vi "PPS TimeKeeper.vi"() -> ()   [LabVIEW 2016]
uses:
  LockPPS_State.ctl
  <vilib>/Platform/TimedLoop/XDataNode/timing_clust.ctl
  <vilib>/Platform/TimedLoop/XDataNode/nitl_modes.ctl
  <vilib>/Platform/TimedLoop/XDataNode/wakeup.ctl
  <vilib>/rvi/Emulation/niFpgaSctlEmulationGetInTimedLoop.vi
  <vilib>/rvi/Emulation/niFpgaEmulationReportErrorSimple.vi
  <vilib>/rvi/Emulation/niFpgaGetClockAttributes.vi
  <vilib>/rvi/Emulation/niFpgaCriticalErrorInLSC.vi
  <vilib>/rvi/eio/common/nirviEmuTemplateMethod_errors.vi
  <vilib>/Platform/TimedLoop/XDataNode/XDataNode.xnode
  <vilib>/eio/EIONode/EIONode.xnode
  <vilib>/rvi/FXPMathLib/basic elements/FxpDiscreteDelay/XNode/nifxpmath_DiscreteDelay.xnode
  <vilib>/Platform/TimedLoop/XDataNode/XDNodeRunTimeDep.lvlib
  <instrlib>/_niInstr/Basic Elements/v1/FPGA/niInstr Basic Elements v1 FPGA.lvlib
panel:
  out "state":T1
  in  "Dleay":u16=500
  out "PPS":u64
  in  "Period":u64=100000000 format="%.0p"
  in  "Lock":bool
  out "Time-ns":u64 format="%.0p"
  in  "Sync Counter Load Val":u64 format="%.0p"
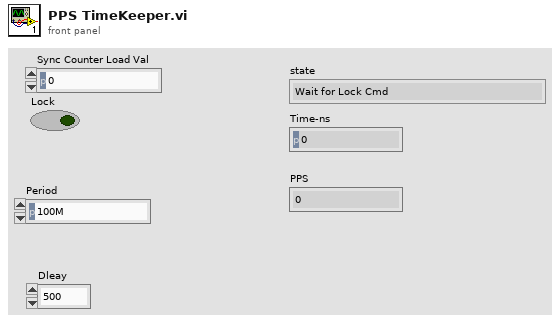
[diagram p1: front panel]
types:
  T1 = typedef "LockPPS_State.ctl" = enum16{"Wait for Lock Cmd", "Wait for PPS"}
  T2 = typedef "XDNodeRunTimeDep.lvlib/timing_clust.ctl" = cluster{"Expected End [f-1]":u64, "Actual End [f-1]":u64, "Finished Late? [f-1]":bool, "Expected End [i-1]":u64, "Actual End [i-1]":u64, "Finished Late? [i-1]":bool, "Expected Start [i]":u64, "Actual Start [i]":u64, "Expected Start [f]":u64, "Actual Start [f]":u64, "Source Name":string, "Structure Name":string, "Period":i64, "Deadline":i64, "Offset":i64, "Start":i64, "Priority":i32, "Timeout":i32, "Mode":T3, "Wakeup Reason":T4, "Error":errorcluster, "Source Type":string, "Secondary Source Type":string, "Global End Time":u64, "Global Start Time":u64, "Frame Duration":u64, "Iteration Duration":u64, "Assigned CPU":i32, "I/O Scan Engine Mode":u32}
  T3 = typedef "XDNodeRunTimeDep.lvlib/nitl_modes.ctl" = enum32{"No Change", "Process missed periods, maintain original phase", "Discard missed periods, maintain original phase", "Process missed periods, ignore original phase", "Discard missed periods, ignore original phase"}
  T4 = typedef "XDNodeRunTimeDep.lvlib/wakeup.ctl" = enum32{"Normal", "Aborted", "Asynchronous wakeup", "Timing source error", "Timed loop error", "Timeout"}
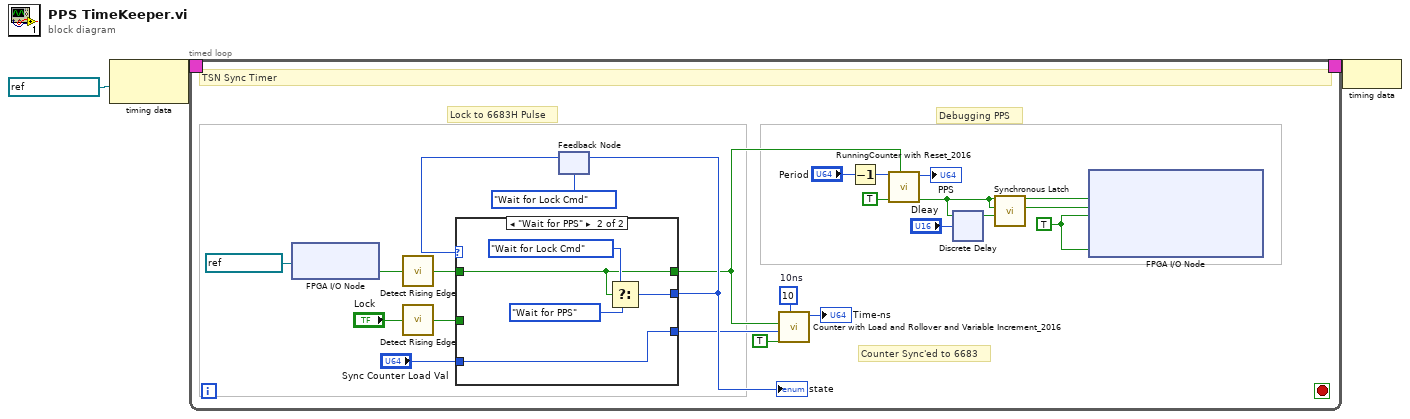
[diagram p0: block diagram]
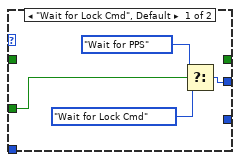
[diagram p2: hidden frame]
diagram:
  n1 = node-c288(refnum<k21> "PXIe_Clk100" ("Source Name")) -> (w3:T2)
  n2 = timed-loop {
    timing: w3 -> [_]
    timing-out: [_] -> w2
    stop <- _ stop-if-true
    w7 = u64 10  # 10ns
    w11 = TRUE ("Ethernet\\PFI0_OutEnable")
    # "Counter Sync'ed to 6683"
    # "Lock to 6683H Pulse"
    # "Debugging PPS"
    # "TSN Sync Timer"
    n3 = xnode "FPGA I/O Node"("FPGA I/O In"=refnum<k21> "PXI_Trig7") -> ("I/O Item"=w19:bool)  [unwired: 1 out]
    n4 = call <instrlib>:"Detect Rising Edge.vi"("signal"=w19) -> ("edge detected"=w20:bool)  [unwired: 14 in]
    n5 = call <instrlib>:"Detect Rising Edge.vi"("signal"="Lock") -> ("edge detected"=w25:bool)  [unwired: 14 in]
    n6 = feedback #1(LockPPS_State."Wait for Lock Cmd") -> (w23:T1)
    n7 = case shown="\"Wait for PPS\"" w23 {
      tunnel: w25 -> [w30 _]
      tunnel: [w27 w31] -> w24
      tunnel: w20 -> [_ w33]
      tunnel: [_ w33] -> w6
      tunnel: "Sync Counter Load Val" -> [_ w35]
      tunnel: [_ w35] -> w9
      frame "Wait for Lock Cmd", Default {
        n8 = Select(t=LockPPS_State."Wait for PPS", s=w30, f=LockPPS_State."Wait for Lock Cmd") -> (s? t:f=w27:T1)
      }
      frame "Wait for PPS" {
        n9 = Select(t=LockPPS_State."Wait for Lock Cmd", s=w33, f=LockPPS_State."Wait for PPS") -> (s? t:f=w31:T1)
      }
    }
    "state" <- w24
    n10 = feedback-in #1(w24) -> ()
    n11 = call "Counter with Load and Rollover and Variable Increment_2016.vi"("Increment"=w7, "INC?"=TRUE, "Load Value"=w9, "Load?"=w6) -> ("count"=→"Time-ns":u64)  [unwired: 7 in]
    n12 = Decrement(x="Period") -> (x-1=w17:u64)
    n13 = call "RunningCounter with Reset_2016.vi"("Reset?"=w6, "INC?"=TRUE, "rollover"=w17) -> ("rollover"=w14:bool, "count"=→"PPS":u64)  [unwired: 7 in]
    n14 = xnode ("Discrete Delay")("D"=w14, "n-1[0..511]"="Dleay") -> ("Q"=w13:bool)
    n15 = call <instrlib>:"Synchronous Latch.vi"("clear"=w13, "set"=w14) -> ("out"=w12:bool)  [unwired: 9 in]
    n16 = xnode "FPGA I/O Node"("Ethernet\\PFI0_Out"=w14, "Ethernet\\PFI0_OutEnable"=w11, "Ethernet\\PFI1_Out"=w12, "Ethernet\\PFI1_OutEnable"=w11) -> ()  [unwired: 4 in, 4 out]
  }
  n17 = node-c288(w2) -> ()
